vi "Cluster.vi"() -> ()   [LabVIEW 2021]
panel:
  out "Cluster Modified":T1
  out "output cluster":cluster{"Boolean 2":bool, "Slide":dbl}
  out "Slide":dbl
  out "Boolean 2":bool
  out "Boolean":bool
  out "Numeric":dbl
  in  "Cluster 3":T1 {"Slide" scale=0.0..10.0}
  out "Direct Conection Out":T1 {"Slide" scale=0.0..10.0}
  in  "Direct Conection In":T1 {"Slide" scale=0.0..10.0}
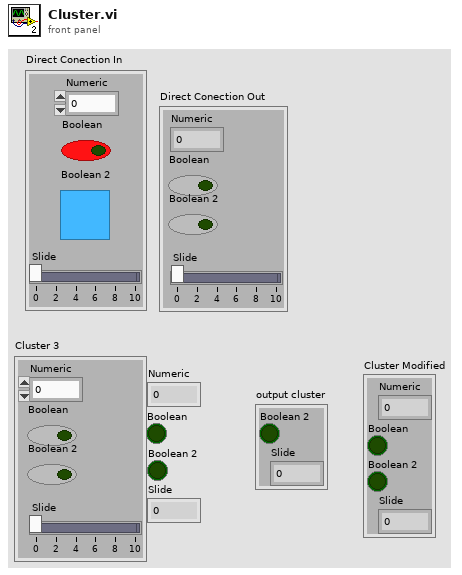
[diagram p1: front panel]
types:
  T1 = cluster{"Numeric":dbl, "Boolean":bool, "Boolean 2":bool, "Slide":dbl}
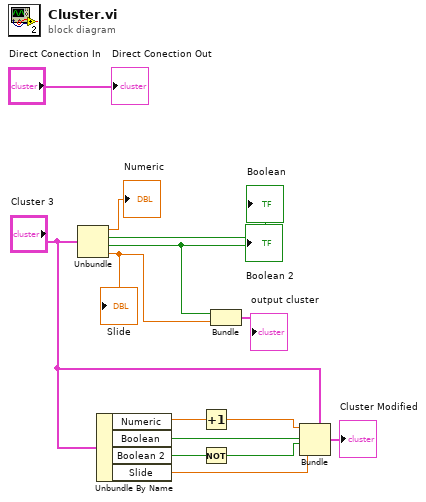
[diagram p0: block diagram]
diagram:
  n1 = Unbundle("Cluster 3") -> ("Numeric"=→"Numeric":dbl, "Boolean"=→"Boolean":bool, "Boolean 2"=w11:bool, "Slide"=w10:dbl)
  "Boolean 2" <- w11
  "Slide" <- w10
  n2 = Unbundle By Name("Cluster 3") -> ("Numeric"=w7:dbl, "Boolean"=w4:bool, "Boolean 2"=w8:bool, "Slide"=w2:dbl)
  n3 = Increment(x=w7) -> (x+1=w5:dbl)
  n4 = Not(x=w8) -> (.not. x?=w3:bool)
  n5 = Bundle("Boolean 2"=w11, "Slide"=w10) -> (→"output cluster":cluster{"Boolean 2":bool, "Slide":dbl})  [unwired: 1 in]
  n6 = Bundle(cluster="Cluster 3", "Numeric"=w5, "Boolean"=w4, "Boolean 2"=w3, "Slide"=w2) -> (→"Cluster Modified":T1)
  "Direct Conection Out" <- "Direct Conection In"
